vi "Receive Datum Update.vi"(8 "Publication Time":timestamp, 9 "Value":variant, 10 "Datum Name":string, 11 "ListboxBusMonitorPanel in":refnum<class "ListboxBusMonitorPanel.lvclass">) -> (3 "ListboxBusMonitorPanel out":refnum<class "ListboxBusMonitorPanel.lvclass">)   [LabVIEW 2017, in "ListboxBusMonitor.lvlib" / "ListboxBusMonitorPanel.lvclass"]
uses:
  ListboxBusMonitorPanel.lvclass
  ListboxBusMonitorPanel.lvclass/ListboxBusMonitorPanel.ctl
  gpm_packages/@cs/variant/Source/Format Value String.vi
  gpm_packages/@cs/variant/Source/Scalar Data to String.vi
  <vilib>/Utility/Data Type/Get Type Information.vi
  <vilib>/Utility/Data Type/Get Refnum Information.vi
  gpm_packages/@cs/variant/Source/Format Type String.vi
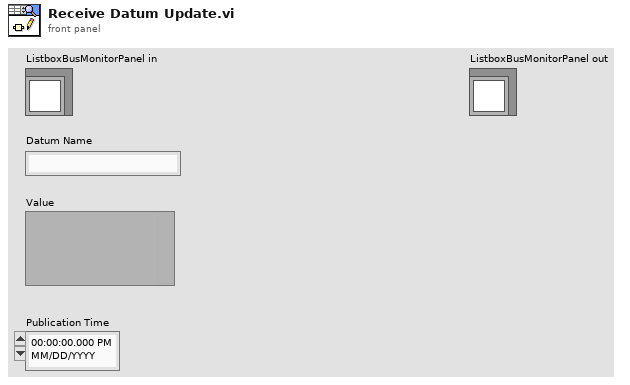
[diagram p1: front panel]
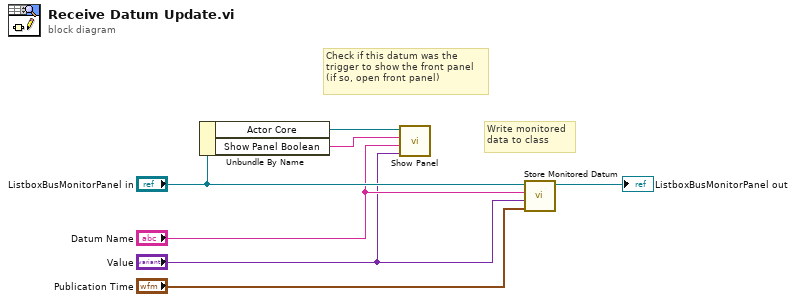
[diagram p0: block diagram]
diagram:
  # "Write monitored\ndata to class"
  # "Check if this datum was the\ntrigger to show the front panel\n(if so, open front panel)"
  n1 = Unbundle By Name("ListboxBusMonitorPanel in") -> ("Actor Core"=w7:refnum<vi>, "Show Panel Boolean"=w4:string)
  n2 = call "Show Panel.vi"("Value"="Value", "Datum Name"="Datum Name", "Show Panel Boolean"=w4, "VI in"=w7) -> ()  [unwired: 8 in]
  n3 = call "Store Monitored Datum.vi"("Publication Time"="Publication Time", "Value"="Value", "Datum Name"="Datum Name", "ListboxBusMonitorPanel in"="ListboxBusMonitorPanel in") -> ("ListboxBusMonitorPanel out"=→"ListboxBusMonitorPanel out":refnum<class "ListboxBusMonitorPanel.lvclass">)  [unwired: 7 in]
